vi "Quick Usb Get String Descriptor.vi"(7 "length":u16, 8 "error in (no error)":errorcluster, 9 "buffer":string, 10 "index":u8, 11 "hDevice":u32) -> (0 "error out":errorcluster, 1 "buffer out":string, 2 "function return":i32, 3 "hDevice out":u32)   [LabVIEW 2011, in "QuickUSB.lvlib"]
doc: "QUSBLIB QRETURN QuickUsbGetStringDescriptor(\n QHANDLE hDevice, \n QBYTE index,\n PQCHAR buffer, \n QWORD length\n);"
uses:
  QuickUSB.lvlib
  QuickUSB.dll
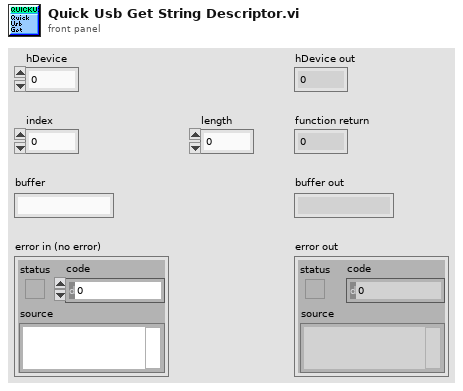
[diagram p1: front panel]
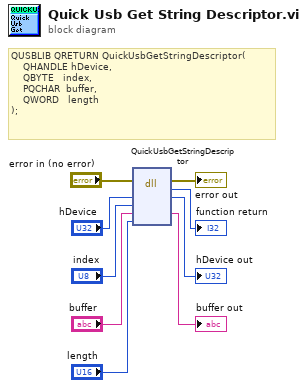
[diagram p0: block diagram]
diagram:
  # "QUSBLIB QRETURN QuickUsbGetStringDescriptor(\n    QHANDLE hDevice, \n    QBYTE   index,\n    PQCHAR  buffer, \n    QWORD   length\n);"
  n1 = dll-call lib="C:/QuickUSB/QuickUSB.*" fn="QuickUsbGetStringDescriptor"(error in="error in (no error)", "hDevice"="hDevice", "index"="index", "buffer"="buffer", "length"="length") -> (error out=→"error out":errorcluster, →"function return":i32, "hDevice"=→"hDevice out":u32, "buffer"=→"buffer out":string)  [unwired: 4 in, 1 out]
